vi "Sweep magnet.vi"() -> ()   [LabVIEW 2021]
panel:
  in  "Wait (min)":dbl[](array[numeric])
  in  "Rate (T/min)":dbl[](array[numeric])
  in  "H (T)":dbl[](array[numeric])
  # "The Sweepificator"
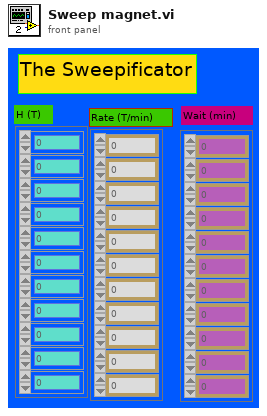
[diagram p1: front panel]
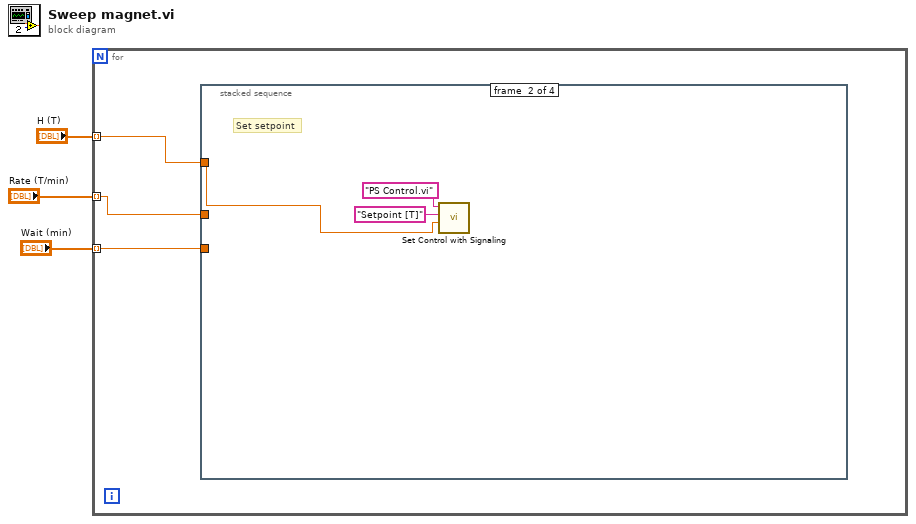
[diagram p0: block diagram]
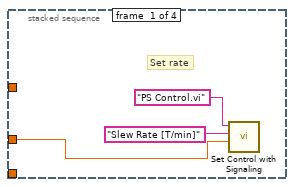
[diagram p2: hidden frame]
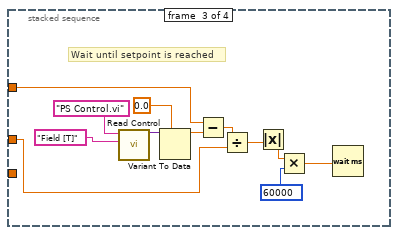
[diagram p3: hidden frame]
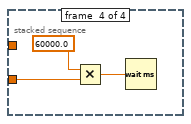
[diagram p4: hidden frame]
diagram:
  n1 = for {
    tunnel: "H (T)" -> [w6] mode=indexing
    tunnel: "Rate (T/min)" -> [w5] mode=indexing
    tunnel: "Wait (min)" -> [w4] mode=indexing
    n2 = stacked-sequence {
      tunnel: w6 -> [_ w11 w22 _]
      tunnel: w5 -> [w7 _ w20 _]
      tunnel: w4 -> [_ _ _ w27]
      frame #0 {
        # "Set rate"
        n3 = call "Set Control with Signaling.vi"("Value"=w7, "Control Name"="Slew Rate [T/min]", "VI Name"="PS Control.vi") -> ()  [unwired: 8 in, 1 out]
      }
      frame #1 {
        # "Set setpoint"
        n4 = call "Set Control with Signaling.vi"("Value"=w11, "Control Name"="Setpoint [T]", "VI Name"="PS Control.vi") -> ()  [unwired: 8 in, 1 out]
      }
      frame #2 {
        # "Wait until setpoint is reached"
        n5 = call "Read Control.vi"("VI Name"="PS Control.vi", "Control Name"="Field [T]") -> ("Value"=w15:variant)  [unwired: 3 in, 1 out]
        n6 = Variant To Data(type=0.0 ("Numeric"), Variant=w15) -> (data=w14:dbl)  [unwired: 1 in, 1 out]
        n7 = Subtract(x=w22, y=w14) -> (x-y=w21:dbl)
        n8 = Divide(x=w21, y=w20) -> (x/y=w19:dbl)
        n9 = Absolute Value(x=w19) -> (abs(x)=w18:dbl)
        n10 = Multiply(x=w18, y=60000) -> (x*y=w16:dbl)
        n11 = Wait (ms)(milliseconds to wait=w16) -> ()  [unwired: 1 out]
      }
      frame #3 {
        n12 = Multiply(x=60000.0, y=w27) -> (x*y=w26:dbl)
        n13 = Wait (ms)(milliseconds to wait=w26) -> ()  [unwired: 1 out]
      }
    }
  }
